vi "Destroy.vi"(8 "error in (no error)":errorcluster, 11 "Asteroid in":refnum<class "Asteroid.lvclass">) -> (0 "error out":errorcluster)   [LabVIEW 2021, in "Asteroid.lvclass"]
uses:
  Asteroid.lvclass
  Asteroid.lvclass/Asteroid.ctl
  Resource Manager/Resource Manager.lvclass
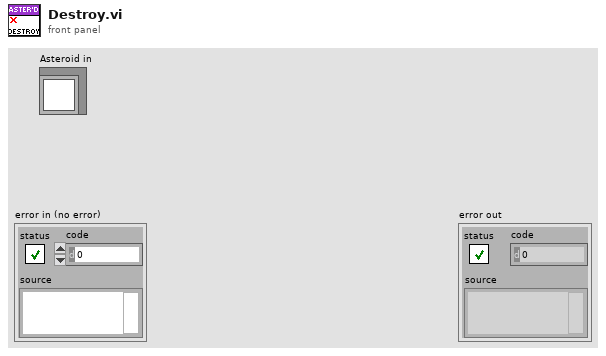
[diagram p1: front panel]
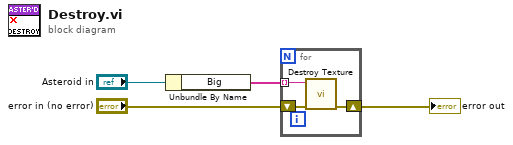
[diagram p0: block diagram]
diagram:
  n1 = Unbundle By Name("Asteroid in") -> ("Big"=w2:string[])
  n2 = for {
    shift-right: [w6] -> w3
    shift-left: "error in (no error)" -> [w7]
    tunnel: w2 -> [w5] mode=indexing
    n3 = call "Destroy Texture.vi"("error in (no error)"=w7, "Texture Name"=w5) -> ("error out"=w6:errorcluster)  [unwired: 9 in]
  }
  "error out" <- w3
